vi "F Dwf Digital Spi Select.vi"(8 "error in (no error)":errorcluster, 9 "level":i32, 10 "idxChannel":i32, 11 "hdwf":i32) -> (0 "error out":errorcluster, 3 "function return":i32)   [LabVIEW 2021, in "Olasdwf.lvlib"]
doc: "DWFAPI int FDwfDigitalSpiSelect(HDWF hdwf, int idxChannel, int level);"
uses:
  Olasdwf.lvlib
  Windows/System32/dwf.dll
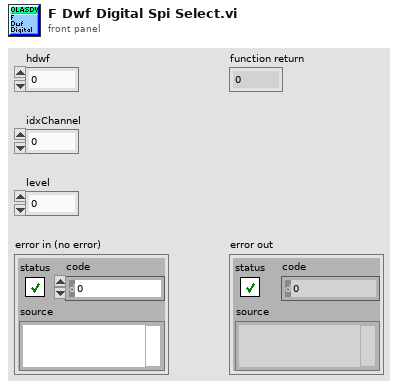
[diagram p1: front panel]
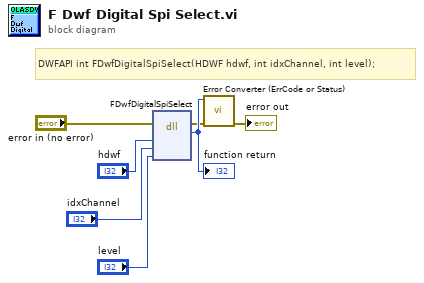
[diagram p0: block diagram]
diagram:
  # "DWFAPI int FDwfDigitalSpiSelect(HDWF hdwf, int idxChannel, int level);"
  n1 = dll-call lib="/Windows/System32/dwf.*" fn="FDwfDigitalSpiSelect"(error in="error in (no error)", "hdwf"="hdwf", "idxChannel"="idxChannel", "level"="level") -> (error out=w2:errorcluster, w7:i32)  [unwired: 5 in, 1 out]
  "function return" <- w7
  n2 = call "Error Converter (ErrCode or Status).vi"("error in (no error)"=w2, "error code"=w7) -> ("error out"=→"error out":errorcluster)  [unwired: 9 in]
